vi "Example_hello_world.vi"() -> ()   [LabVIEW 8.6]
panel:
  out "error out":errorcluster
  out "function return 2":string
  # "hello_world.xlsx"
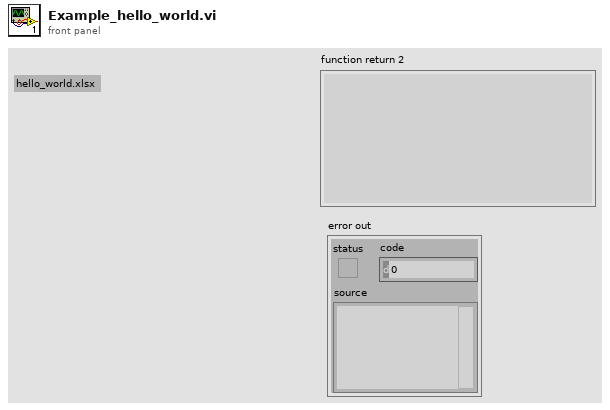
[diagram p1: front panel]
types:
  T1 = enum32{"invalid app kind", "Development System", "Run Time System", "Student Edition", "Embedded LabVIEW", "Evaluation", "Custom"}
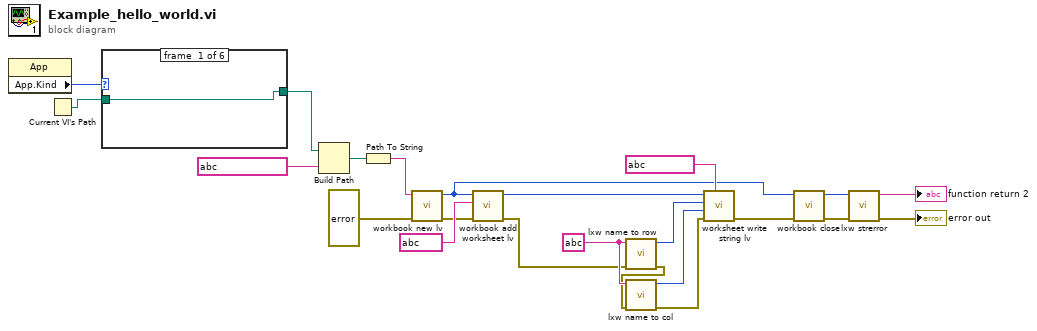
[diagram p0: block diagram]
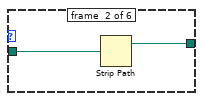
[diagram p2: hidden frame]
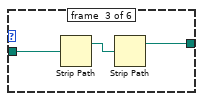
[diagram p3: hidden frame]
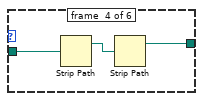
[diagram p4: hidden frame]
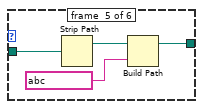
[diagram p5: hidden frame]
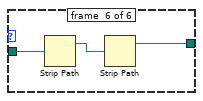
[diagram p6: hidden frame]
diagram:
  w17 = string ? ("row_str")
  n1 = property class="App"() -> ("App.Kind"=w23:T1)  [unwired: 2 in, 2 out]
  n2 = Current VI's Path() -> (path=w22:path)
  n3 = case shown="\"Evaluation\"" w23 {
    tunnel: w22 -> [w24 w26 w29 w32 w36 w39]
    tunnel: [w24 w25 w27 w30 w34 w37] -> w21
    frame #0 {
    }
    frame #1 {
      n4 = Strip Path(path=w26) -> (stripped path=w25:path)  [unwired: 1 out]
    }
    frame #2 {
      n5 = Strip Path(path=w29) -> (stripped path=w28:path)  [unwired: 1 out]
      n6 = Strip Path(path=w28) -> (stripped path=w27:path)  [unwired: 1 out]
    }
    frame #3 {
      n7 = Strip Path(path=w32) -> (stripped path=w31:path)  [unwired: 1 out]
      n8 = Strip Path(path=w31) -> (stripped path=w30:path)  [unwired: 1 out]
    }
    frame #4 {
      n9 = Strip Path(path=w36) -> (stripped path=w35:path)  [unwired: 1 out]
      n10 = Build Path(base path=w35, name or relative path=string ?) -> (appended path=w34:path)
    }
    frame #5 {
      n11 = Strip Path(path=w39) -> (stripped path=w38:path)  [unwired: 1 out]
      n12 = Strip Path(path=w38) -> (stripped path=w37:path)  [unwired: 1 out]
    }
  }
  n13 = Build Path(base path=w21, name or relative path=string ? ("filename")) -> (appended path=w2:path)
  n14 = Path To String(path=w2) -> (string=w1:string)
  n15 = call "workbook new lv.vi"("error in (no error)"=errorcluster ?, "filename"=w1) -> ("error out"=w14:errorcluster, "function return"=w3:u32)  [unwired: 8 in]
  n16 = call "workbook add worksheet lv.vi"("error in (no error)"=w14, "sheetname"=string ?, "workbook"=w3) -> ("error out"=w12:errorcluster, "function return"=w18:u32)  [unwired: 7 in]
  n17 = call "lxw name to row.vi"("error in (no error)"=w12, "row_str"=w17) -> ("error out"=w11:errorcluster, "function return"=w16:u32)  [unwired: 8 in]
  n18 = call "lxw name to col.vi"("error in (no error)"=w11, "col_str"=w17) -> ("error out"=w10:errorcluster, "function return"=w15:u16)  [unwired: 8 in]
  n19 = call "worksheet write string lv.vi"("string"=string ?, "error in (no error)"=w10, "col"=w15, "row"=w16, "worksheet"=w18) -> ("error out"=w5:errorcluster)  [unwired: 5 in, 1 out]
  n20 = call "workbook close.vi"("error in (no error)"=w5, "workbook"=w3) -> ("error out"=w6:errorcluster, "function return"=w8:u32)  [unwired: 8 in]
  n21 = call "lxw strerror.vi"("error in (no error)"=w6, "error_num"=w8) -> ("error out"=→"error out":errorcluster, "function return"=→"function return 2":string)  [unwired: 8 in]
